vi "XW calib mesh and tree checker_PN.vi"() -> ()   [LabVIEW 2010]
uses:
  <vilib>/Utility/miscctls.llb/LVBoundsTypeDef.ctl
  Trimmed down TreeNode2D.ctl
panel:
  out "Status":string="Status report will be presented here"
  out "Null-zone check (ensure there are no gray areas within the triangle mesh)":picture
  in  "Viewport size (pix)":u32=720
  in  "Highlight mesh and tree":bool=TRUE
  out "Tri-mesh":picture
  out "Interactive mode ready":bool
  out "E2 (Volts)":dbl
  out "E1 (Volts)":dbl
  out "V (m/s)":dbl=nan
  out "U (m/s)":dbl=nan
  out "Voltages are inside calibrated region":bool
  in  "Stop interactive mode":bool
  out "Tree":picture
  out "Node stack size history":i32[](graph)
  out "All nodes processed and processed without error":bool
  in  "Sf":dbl=0.6
  in  "dq":dbl=0.3927
  in  "L0":dbl=1.0
  in  "Pad":dbl=1.01
  in  "XW_Calib_Map file path (dialog if empty)":path=path "C:/Documents and Settings/Paul Nathan/Desktop/XW Calib Map/XW Calib Map TRIMESH vi/XW_Map_Wire001OH65_080210.txt"
  # "Paul Nathan 07/03/10"
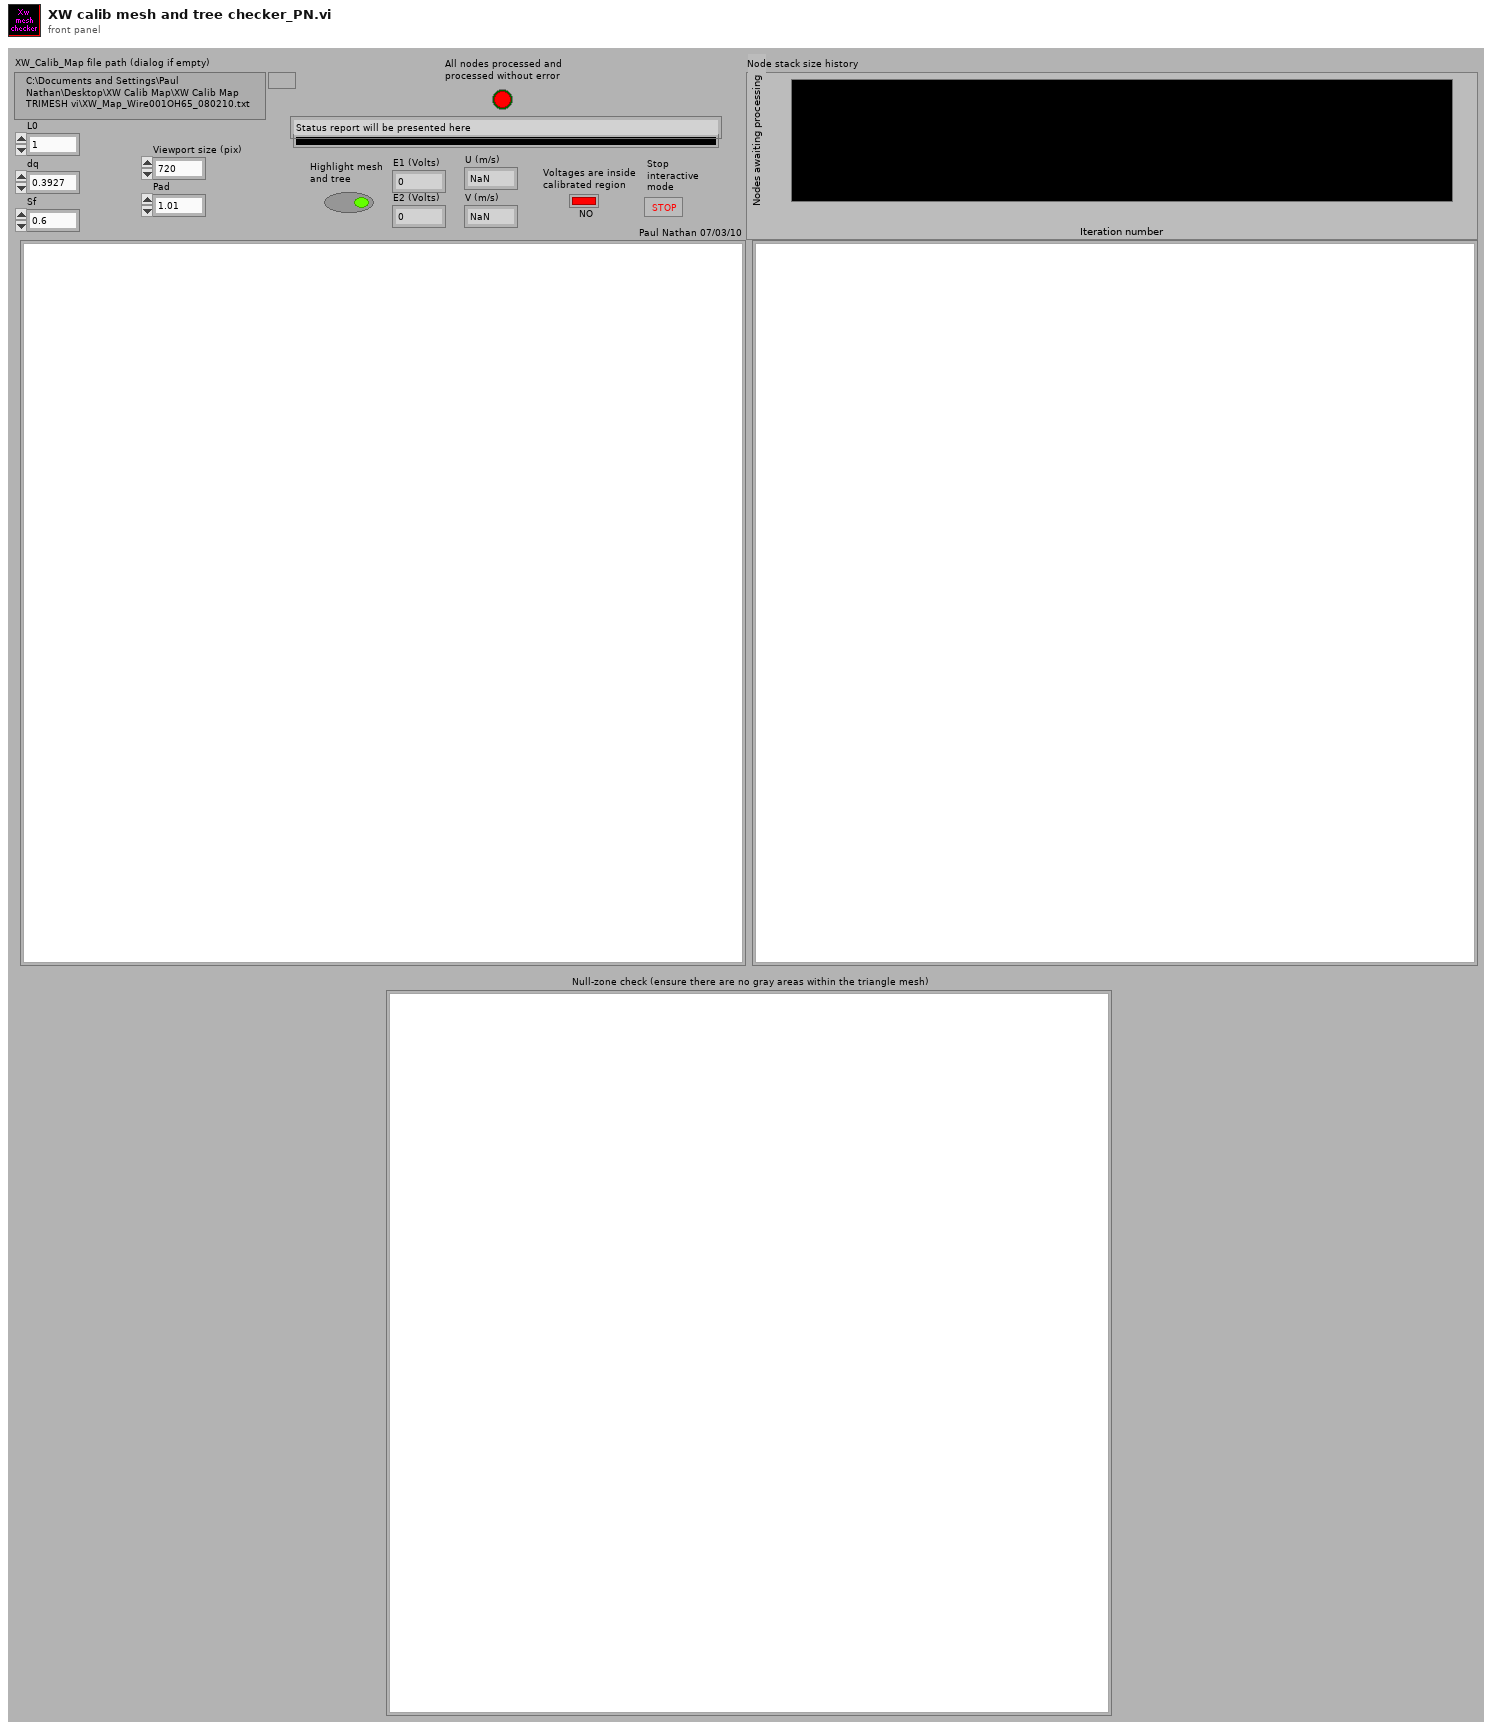
[diagram p1: front panel]
types:
  T1 = typedef "LVBoundsTypeDef.ctl" = cluster{"Width":u32, "Height":u32}
  T2 = cluster{"Width":i16, "Style":enum32{"Solid", "Dash", "Dot", "DashDot", "DashDotDot"}}
  T3 = cluster{"Width":u16, "Style":enum32{"Solid", "Dash", "Dot", "DashDot", "DashDotDot"}}
  T4 = typedef "Trimmed down TreeNode2D.ctl" = cluster{"Xmax":dbl, "Xmin":dbl, "Ymax":dbl, "Ymin":dbl, "Xc":dbl, "Yc":dbl, "ObjIndexList":i32[], "NodeQ1Index":i32, "NodeQ2Index":i32, "NodeQ3Index":i32, "NodeQ4Index":i32}
  T5 = typedef "Triangle2D.ctl" = cluster{"V10":dbl[], "V20":dbl[], "1/det":dbl, "V0":cluster{"PosVector":dbl[], "ValueVector":dbl[]}, "V1":cluster{"PosVector":dbl[], "ValueVector":dbl[]}, "V2":cluster{"PosVector":dbl[], "ValueVector":dbl[]}, "V21":dbl[]}
  T6 = cluster{"Xmax":dbl, "Xmin":dbl, "Ymax":dbl, "Ymin":dbl}
  T7 = typedef "TreeNode2D.ctl" = cluster{"Xmax":dbl, "Xmin":dbl, "Ymax":dbl, "Ymin":dbl, "Xc":dbl, "Yc":dbl, "Px":dbl, "Py":dbl, "q":dbl, "Level":i32, "ObjIndexList":i32[], "ParentIndex":i32, "NodeQ1Index":i32, "NodeQ2Index":i32, "NodeQ3Index":i32, "NodeQ4Index":i32, "EdgeVectorsQ1":dbl[][], "EdgeVectorsQ2":dbl[][], "EdgeVectorsQ3":dbl[][], "EdgeVectorsQ4":dbl[][], "PointOnEdgeVectorsQ1":dbl[][], "PointOnEdgeVectorsQ2":dbl[][], "PointOnEdgeVectorsQ3":dbl[][], "PointOnEdgeVectorsQ4":dbl[][]}
  T8 = typedef "LVMouseTypeDef.ctl" = cluster{"Mouse Position":cluster{"X":i32, "Y":i32}, "Mouse Modifiers":cluster{"Button Down":bool, "Shift Mod":bool, "Menu Mod":bool, "Option Mod":bool}}
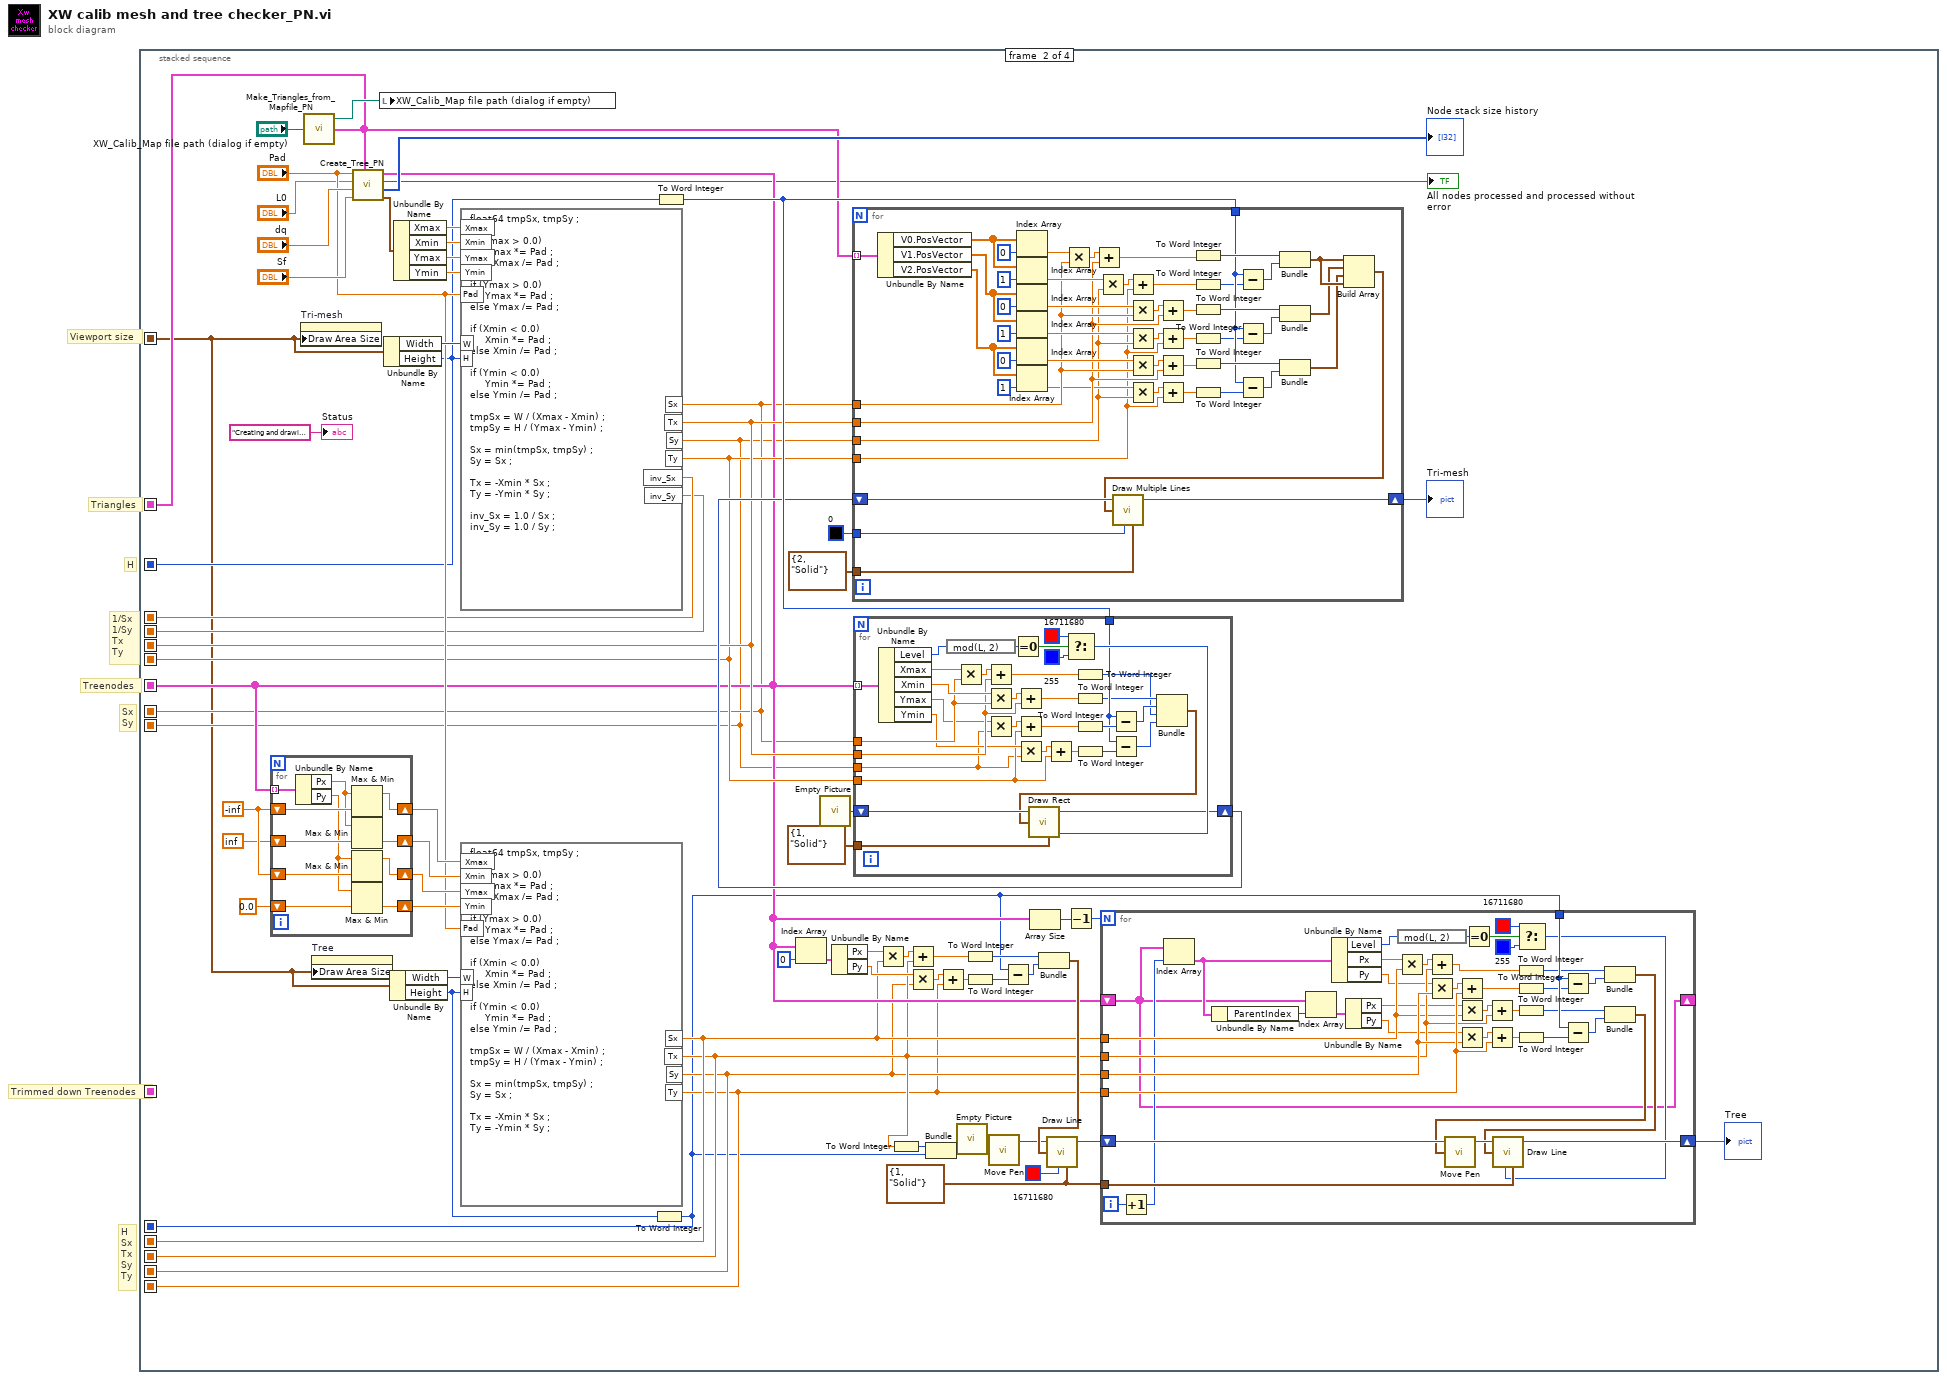
[diagram p0: block diagram]
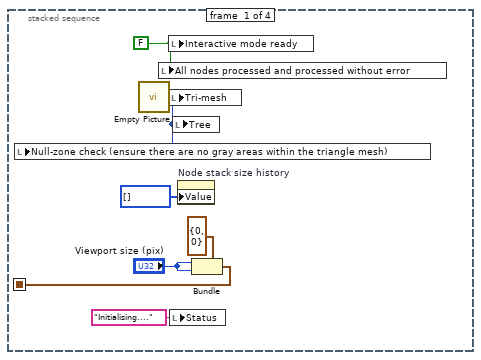
[diagram p2: hidden frame]
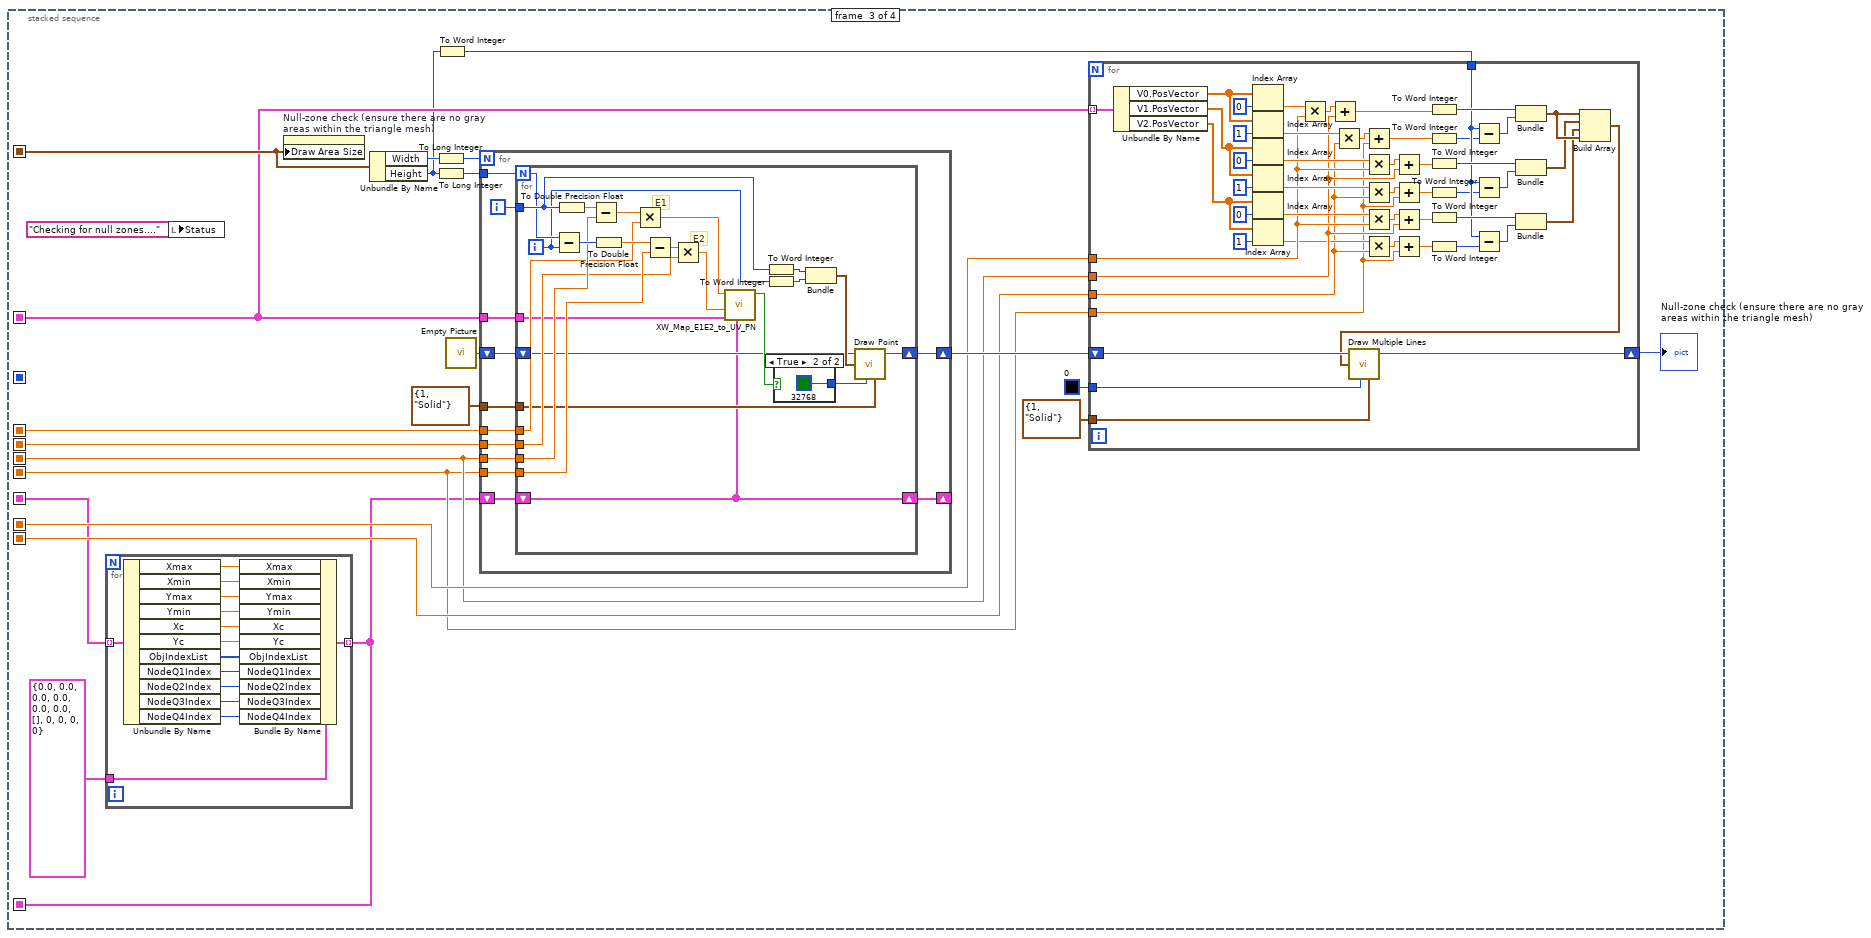
[diagram p3: hidden frame]
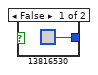
[diagram p4: hidden frame]
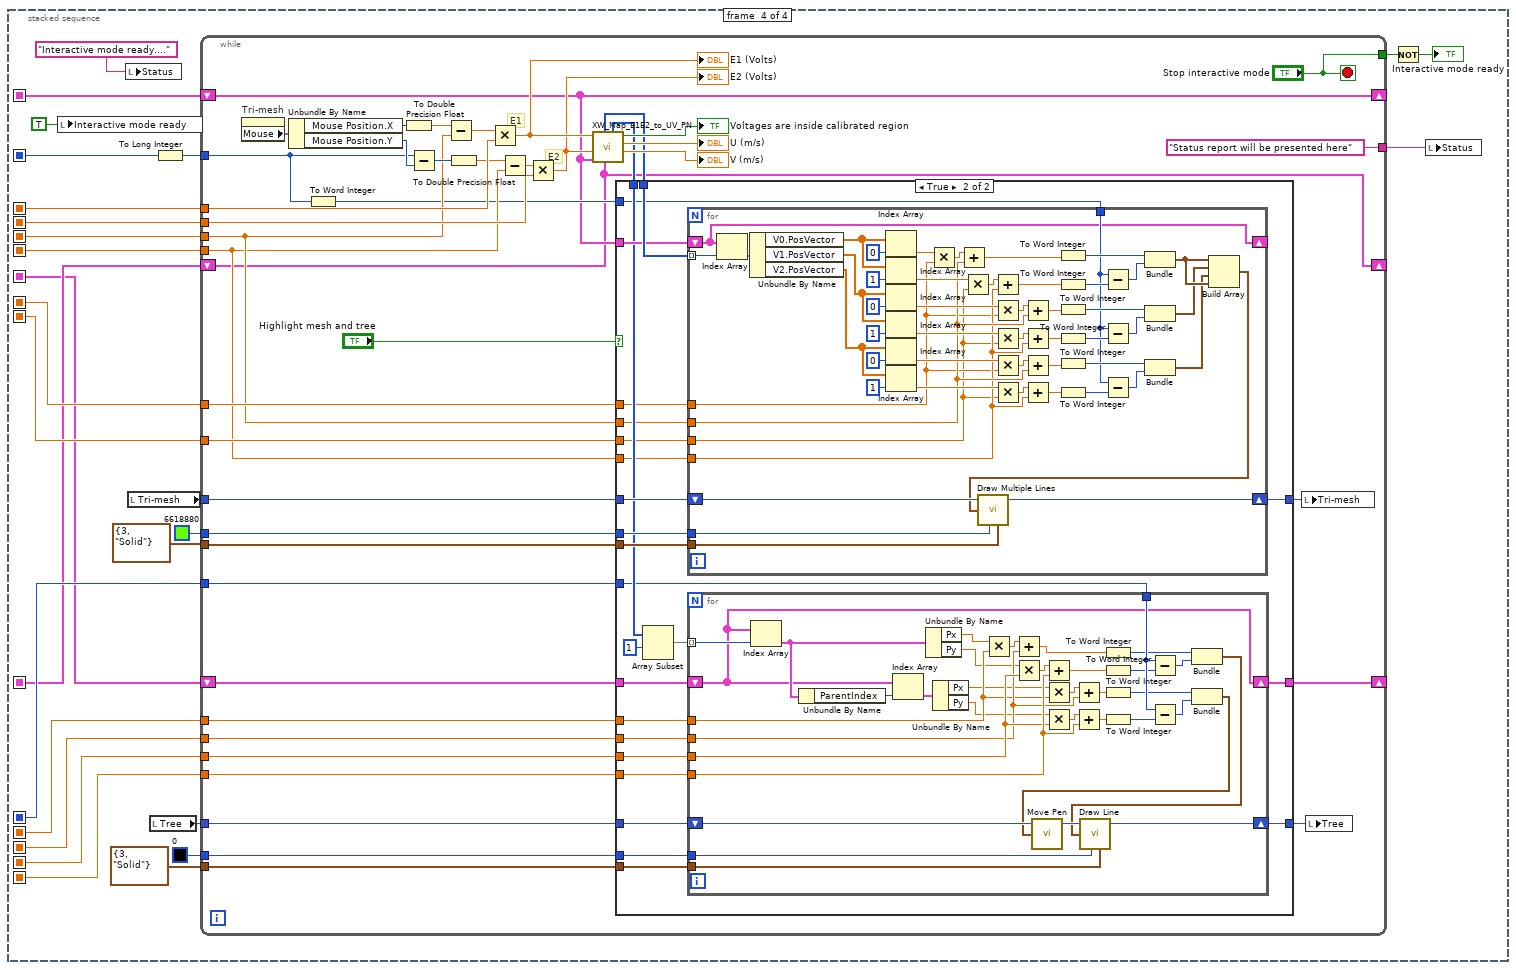
[diagram p5: hidden frame]
diagram:
  # "Trimmed down Treenodes"
  # "Viewport size"
  # "H\nSx\nTx\nSy\nTy"
  # "Sx\nSy"
  # "Treenodes"
  # "Triangles"
  # "H"
  # "1/Sx\n1/Sy\nTx\nTy"
  n1 = stacked-sequence {
    seq-local: [_ w29 _ _] -> [_ _ w230 w354]
    seq-local: [_ w28 _ _] -> [_ _ w229 w353]
    seq-local: [_ w27 _ _] -> [_ _ w219 w363]
    seq-local: [_ w26 _ _] -> [_ _ w218 w362]
    seq-local: [_ w25 _ _] -> [_ _ _ w361]
    seq-local: [_ w22 _ _] -> [_ _ w213 w337]
    seq-local: [_ w24 _ _] -> [_ _ w222 w359]
    seq-local: [_ w19 _ _] -> [_ _ w221 w348]
    seq-local: [_ w18 _ _] -> [_ _ w220 w347]
    seq-local: [_ w12 _ _] -> [_ _ _ w342]
    seq-local: [_ w16 _ _] -> [_ _ _ w346]
    seq-local: [_ w15 _ _] -> [_ _ _ w345]
    seq-local: [_ w14 _ _] -> [_ _ _ w344]
    seq-local: [_ w13 _ _] -> [_ _ _ w343]
    seq-local: [w4 _ _ _] -> [_ w11 w234 _]
    seq-local: [_ _ w212 _] -> [_ _ _ w338]
    frame #0 {
      w2 = FALSE
      n2 = call "Empty Picture"() -> ("empty picture"=w3:picture)
      n3 = local write "Null-zone check (ensure there are no gray areas within the triangle mesh)"(w3) -> ()
      n4 = local write "All nodes processed and processed without error"(w2) -> ()
      n5 = local write "Interactive mode ready"(w2) -> ()
      n6 = local write "Tri-mesh"(w3) -> ()
      n7 = local write "Status"("Initialising....") -> ()
      n8 = local write "Tree"(w3) -> ()
      n9 = property on="Node stack size history" class="WFGraph (strict)"("Value"=i32[] [] ("Node stack size history")) -> ()  [unwired: 2 in, 2 out]
      n10 = Bundle(cluster=T1 {"Width"=0, "Height"=0} ("Draw Area Size"), "Width"="Viewport size (pix)", "Height"="Viewport size (pix)") -> (w4:T1)
    }
    frame #1 {
      w32 = T3 {"Width"=1, "Style"=enum."Solid"} ("pen")
      w53 = -inf
      n11 = property on="Tri-mesh" class="Pict"("Draw Area Size"=w11) -> ()  [unwired: 2 in, 2 out]
      n12 = call "Make_Triangles_from_Mapfile_PN.vi"("XW_Calib_Map file path (dialog if empty)"="XW_Calib_Map file path (dialog if empty)") -> ("XW_Calib_Map file path"=w74:path, "Triangles"=w24:T5[])  [unwired: 1 out]
      n13 = property on="Tree" class="Pict"("Draw Area Size"=w11) -> ()  [unwired: 2 in, 2 out]
      n14 = call "Create_Tree_PN.vi"("Triangles"=w24, "Sf"="Sf", "dq"="dq", "L0"="L0", "Pad"="Pad") -> ("Mesh bounds"=w8:T6, "Node stack size history"=→"Node stack size history":i32[], "All nodes processed and processed without error"=→"All nodes processed and processed without error":bool, "TreeNodes out"=w22:T7[])
      n15 = for {
        shift-right: [w127] -> w55
        shift-left: w53 -> [w125]
        shift-right: [w126] -> w57
        shift-left: w53 -> [w124]
        shift-right: [w122] -> w56
        shift-left: inf -> [w123]
        shift-right: [w120] -> w58
        shift-left: 0.0 -> [w121]
        tunnel: w22 -> [w118] mode=indexing
        n16 = Unbundle By Name(w118) -> ("Px"=w119:dbl, "Py"=w117:dbl)
        n17 = Max & Min(x=w119, y=w125) -> (max(x,y)=w127:dbl)  [unwired: 1 out]
        n18 = Max & Min(x=w119, y=w123) -> (min(x,y)=w122:dbl)  [unwired: 1 out]
        n19 = Max & Min(x=w117, y=w124) -> (max(x,y)=w126:dbl)  [unwired: 1 out]
        n20 = Max & Min(x=w117, y=w121) -> (min(x,y)=w120:dbl)  [unwired: 1 out]
      }
      n21 = local write "XW_Calib_Map file path (dialog if empty)"(w74) -> ()
      n22 = Unbundle By Name(w11) -> ("Width"=w70:u32, "Height"=w25:u32)
      n23 = Unbundle By Name(w11) -> ("Width"=w59:u32, "Height"=w17:u32)
      n24 = Unbundle By Name(w8) -> ("Xmax"=w67:dbl, "Xmin"=w66:dbl, "Ymax"=w65:dbl, "Ymin"=w64:dbl)
      n25 = formula code="float64 tmpSx, tmpSy ;\n\nif (Xmax > 0.0)\n     Xmax *= Pad ;\nelse Xmax /= Pad ;\n\nif (Ymax > 0.0)\n     Ymax *= Pad ;\nelse Ymax /= Pad ;\n\nif (Xmin < 0.0)\n     Xmin *= Pad ;\nelse Xmin /= Pad ;\n\nif (Ymin < 0.0)\n     Ymin *= Pad ;\nelse Ymin /= Pad ;\n\ntmpSx = W / (Xmax - Xmin) ;\ntmpSy = H / (Ymax - Ymin) ;\n\nSx = min(tmpSx, tmpSy) ;\nSy = Sx ;\n\nTx = -Xmin * Sx ;\nTy = -Ymin * Sy ;\n\ninv_Sx = 1.0 / Sx ;\ninv_Sy = 1.0 / Sy ;"("Xmax"=w67, "Xmin"=w66, "Ymax"=w65, "Ymin"=w64, "W"=w70, "H"=w25, "Pad"="Pad") -> ("Sx"=w19:dbl, "Sy"=w18:dbl, "Tx"=w27:dbl, "Ty"=w26:dbl, "inv_Sx"=w29:dbl, "inv_Sy"=w28:dbl)
      n26 = formula code="float64 tmpSx, tmpSy ;\n\nif (Xmax > 0.0)\n     Xmax *= Pad ;\nelse Xmax /= Pad ;\n\nif (Ymax > 0.0)\n     Ymax *= Pad ;\nelse Ymax /= Pad ;\n\nif (Xmin < 0.0)\n     Xmin *= Pad ;\nelse Xmin /= Pad ;\n\nif (Ymin < 0.0)\n     Ymin *= Pad ;\nelse Ymin /= Pad ;\n\ntmpSx = W / (Xmax - Xmin) ;\ntmpSy = H / (Ymax - Ymin) ;\n\nSx = min(tmpSx, tmpSy) ;\nSy = Sx ;\n\nTx = -Xmin * Sx ;\nTy = -Ymin * Sy ;"("Xmax"=w55, "Xmin"=w56, "Ymax"=w57, "Ymin"=w58, "W"=w59, "H"=w17, "Pad"="Pad") -> ("Sx"=w16:dbl, "Sy"=w14:dbl, "Tx"=w15:dbl, "Ty"=w13:dbl)
      n27 = To Word Integer(number=w17) -> (16bit integer=w12:i16)
      n28 = To Word Integer(number=w25) -> (16bit integer=w61:i16)
      n29 = Index Array(array=w22, index=0) -> (element=w48:T7)
      n30 = call "Empty Picture"() -> ("empty picture"=w63:picture)
      n31 = Unbundle By Name(w48) -> ("Px"=w43:dbl, "Py"=w41:dbl)
      n32 = for {
        tunnel: w22 -> [w161] mode=indexing
        tunnel: w19 -> [w146]
        tunnel: w27 -> [w145]
        tunnel: w18 -> [w134]
        tunnel: w26 -> [w136]
        shift-right: [w152] -> w60
        shift-left: w63 -> [w155]
        tunnel: T2 {"Width"=1, "Style"=enum."Solid"} ("pen") -> [w153]
        tunnel: w61 -> [w139]
        n33 = Unbundle By Name(w161) -> ("Level"=w160:i32, "Xmax"=w150:dbl, "Xmin"=w147:dbl, "Ymax"=w142:dbl, "Ymin"=w137:dbl)
        n34 = expression code="mod(L, 2)"(w160) -> (w159:i32)
        n35 = Multiply(x=w150, y=w146) -> (x*y=w151:dbl)
        n36 = Add(x=w151, y=w145) -> (x+y=w149:dbl)
        n37 = Multiply(x=w147, y=w146) -> (x*y=w148:dbl)
        n38 = Multiply(x=w142, y=w134) -> (x*y=w143:dbl)
        n39 = Equal To 0?(x=w159) -> (x = 0?=w158:bool)
        n40 = Add(x=w148, y=w145) -> (x+y=w144:dbl)
        n41 = Add(x=w143, y=w136) -> (x+y=w141:dbl)
        n42 = Multiply(x=w137, y=w134) -> (x*y=w135:dbl)
        n43 = Add(x=w135, y=w136) -> (x+y=w133:dbl)
        n44 = Select(t=u32 16711680, s=w158, f=u32 255) -> (s? t:f=w154:u32)
        n45 = To Word Integer(number=w149) -> (16bit integer=w130:i16)
        n46 = To Word Integer(number=w144) -> (16bit integer=w132:i16)
        n47 = To Word Integer(number=w141) -> (16bit integer=w140:i16)
        n48 = To Word Integer(number=w133) -> (16bit integer=w138:i16)
        n49 = Subtract(x=w139, y=w140) -> (x-y=w131:i16)
        n50 = Subtract(x=w139, y=w138) -> (x-y=w129:i16)
        n51 = Bundle(w132, w131, w130, w129) -> (w128:cluster{i16, i16, i16, i16})  [unwired: 1 out]
        n52 = call <vilib>:"Draw Rect.vi"("picture"=w155, "rect"=w128, "color(black)"=w154, "pen"=w153) -> ("new picture"=w152:picture)  [unwired: 1 in, 4 out]
      }
      n53 = for {
        tunnel: w24 -> [w211] mode=indexing
        shift-right: [w207] -> w23
        shift-left: w60 -> [w208]
        tunnel: u32 0 -> [w210]
        tunnel: T3 {"Width"=2, "Style"=enum."Solid"} ("pen") -> [w209]
        tunnel: w19 -> [w184]
        tunnel: w27 -> [w183]
        tunnel: w18 -> [w180]
        tunnel: w26 -> [w179]
        tunnel: w61 -> [w168]
        n54 = Unbundle By Name(w211) -> ("V0.PosVector"=w197:dbl[], "V1.PosVector"=w196:dbl[], "V2.PosVector"=w195:dbl[])
        n55 = Index Array(array=w197, index=0) -> (element=w194:dbl)
        n56 = Index Array(array=w197, index=1) -> (element=w191:dbl)
        n57 = Index Array(array=w196, index=0) -> (element=w189:dbl)
        n58 = Index Array(array=w196, index=1) -> (element=w187:dbl)
        n59 = Index Array(array=w195, index=0) -> (element=w185:dbl)
        n60 = Index Array(array=w195, index=1) -> (element=w181:dbl)
        n61 = Multiply(x=w194, y=w184) -> (x*y=w193:dbl)
        n62 = Add(x=w193, y=w183) -> (x+y=w175:dbl)
        n63 = Multiply(x=w191, y=w180) -> (x*y=w192:dbl)
        n64 = Add(x=w192, y=w179) -> (x+y=w174:dbl)
        n65 = Multiply(x=w189, y=w184) -> (x*y=w190:dbl)
        n66 = Multiply(x=w187, y=w180) -> (x*y=w188:dbl)
        n67 = Multiply(x=w185, y=w184) -> (x*y=w186:dbl)
        n68 = Multiply(x=w181, y=w180) -> (x*y=w182:dbl)
        n69 = Add(x=w190, y=w183) -> (x+y=w173:dbl)
        n70 = Add(x=w188, y=w179) -> (x+y=w172:dbl)
        n71 = Add(x=w186, y=w183) -> (x+y=w171:dbl)
        n72 = Add(x=w182, y=w179) -> (x+y=w170:dbl)
        n73 = To Word Integer(number=w175) -> (16bit integer=w178:i16)
        n74 = To Word Integer(number=w174) -> (16bit integer=w167:i16)
        n75 = To Word Integer(number=w173) -> (16bit integer=w177:i16)
        n76 = To Word Integer(number=w172) -> (16bit integer=w166:i16)
        n77 = To Word Integer(number=w171) -> (16bit integer=w176:i16)
        n78 = To Word Integer(number=w170) -> (16bit integer=w165:i16)
        n79 = Subtract(x=w168, y=w167) -> (x-y=w164:i16)
        n80 = Subtract(x=w168, y=w166) -> (x-y=w163:i16)
        n81 = Subtract(x=w168, y=w165) -> (x-y=w162:i16)
        n82 = Bundle(w178, w164) -> (w204:cluster{i16, i16})  [unwired: 1 out]
        n83 = Bundle(w177, w163) -> (w201:cluster{i16, i16})  [unwired: 1 out]
        n84 = Bundle(w176, w162) -> (w198:cluster{i16, i16})  [unwired: 1 out]
        n85 = Build Array(w204, w201, w198, w204) -> (w169:cluster{i16, i16}[])
        n86 = call <vilib>:"Draw Multiple Lines.vi"("picture"=w208, "line endpoints"=w169, "color(black)"=w210, "pen"=w209) -> ("new picture"=w207:picture)  [unwired: 1 in, 4 out]
      }
      "Tri-mesh" <- w23
      n87 = Multiply(x=w43, y=w16) -> (x*y=w44:dbl)
      n88 = To Word Integer(number=w15) -> (16bit integer=w47:i16)
      n89 = Add(x=w44, y=w15) -> (x+y=w40:dbl)
      n90 = Multiply(x=w41, y=w14) -> (x*y=w42:dbl)
      n91 = Bundle(w47, w12) -> (w46:cluster{i16, i16})  [unwired: 1 out]
      n92 = Add(x=w42, y=w13) -> (x+y=w39:dbl)
      n93 = call "Empty Picture"() -> ("empty picture"=w45:picture)
      n94 = To Word Integer(number=w40) -> (16bit integer=w37:i16)
      n95 = To Word Integer(number=w39) -> (16bit integer=w38:i16)
      n96 = call <vilib>:"Move Pen.vi"("new position"=w46, "picture"=w45) -> ("new picture"=w34:picture)  [unwired: 1 in, 2 out]
      n97 = Subtract(x=w12, y=w38) -> (x-y=w36:i16)
      n98 = Array Size(array=w22) -> (size(s)=w21:i32)
      n99 = Bundle(w37, w36) -> (w35:cluster{i16, i16})  [unwired: 1 out]
      n100 = call <vilib>:"Draw Line.vi"("picture"=w34, "end point"=w35, "color(black)"=u32 16711680, "pen"=w32) -> ("new picture"=w31:picture)  [unwired: 1 in, 4 out]
      n101 = Decrement(x=w21) -> (x-1=w20:i32)
      n102 = for {
        N: w20 -> [_]
        shift-right: [w115] -> w30
        shift-left: w31 -> [w116]
        tunnel: w32 -> [w113]
        tunnel: w12 -> [w108]
        tunnel: w16 -> [w109]
        tunnel: w15 -> [w110]
        tunnel: w14 -> [w111]
        tunnel: w13 -> [w112]
        shift-right: [w76] -> _
        shift-left: w22 -> [w76]
        i -> [w79]
        n103 = Increment(x=w79) -> (x+1=w78:i32)
        n104 = Index Array(array=w76, index=w78) -> (element=w77:T7)
        n105 = Unbundle By Name(w77) -> ("ParentIndex"=w114:i32)
        n106 = Index Array(array=w76, index=w114) -> (element=w107:T7)
        n107 = Unbundle By Name(w77) -> ("Level"=w102:i32, "Px"=w98:dbl, "Py"=w94:dbl)
        n108 = Unbundle By Name(w107) -> ("Px"=w92:dbl, "Py"=w89:dbl)
        n109 = Multiply(x=w98, y=w109) -> (x*y=w99:dbl)
        n110 = expression code="mod(L, 2)"(w102) -> (w103:i32)
        n111 = Add(x=w99, y=w110) -> (x+y=w97:dbl)
        n112 = Multiply(x=w94, y=w111) -> (x*y=w95:dbl)
        n113 = Add(x=w95, y=w112) -> (x+y=w91:dbl)
        n114 = Multiply(x=w92, y=w109) -> (x*y=w93:dbl)
        n115 = Multiply(x=w89, y=w111) -> (x*y=w90:dbl)
        n116 = Equal To 0?(x=w103) -> (x = 0?=w104:bool)
        n117 = Add(x=w93, y=w110) -> (x+y=w88:dbl)
        n118 = Add(x=w90, y=w112) -> (x+y=w87:dbl)
        n119 = To Word Integer(number=w97) -> (16bit integer=w96:i16)
        n120 = To Word Integer(number=w91) -> (16bit integer=w83:i16)
        n121 = To Word Integer(number=w88) -> (16bit integer=w86:i16)
        n122 = To Word Integer(number=w87) -> (16bit integer=w82:i16)
        n123 = Select(t=u32 16711680, s=w104, f=u32 255) -> (s? t:f=w101:u32)
        n124 = Subtract(x=w108, y=w83) -> (x-y=w85:i16)
        n125 = Subtract(x=w108, y=w82) -> (x-y=w84:i16)
        n126 = Bundle(w96, w85) -> (w80:cluster{i16, i16})  [unwired: 1 out]
        n127 = Bundle(w86, w84) -> (w81:cluster{i16, i16})  [unwired: 1 out]
        n128 = call <vilib>:"Move Pen.vi"("new position"=w81, "picture"=w116) -> ("new picture"=w100:picture)  [unwired: 1 in, 2 out]
        n129 = call <vilib>:"Draw Line.vi"("picture"=w100, "end point"=w80, "color(black)"=w101, "pen"=w113) -> ("new picture"=w115:picture)  [unwired: 1 in, 4 out]
      }
      "Tree" <- w30
      "Status" <- "Creating and drawing mesh, spatial hierarchy and address tree...."
    }
    frame #2 {
      n130 = for {
        tunnel: w213 -> [w248] mode=indexing
        tunnel: [w246] -> w212 mode=indexing
        tunnel: T4 {"Xmax"=0.0, "Xmin"=0.0, "Ymax"=0.0, "Ymin"=0.0, "Xc"=0.0, "Yc"=0.0, "ObjIndexList"=[], "NodeQ1Index"=0, "NodeQ2Index"=0, "NodeQ3Index"=0, "NodeQ4Index"=0} ("Trimmed down TreeNode") -> [w247]
        n131 = Unbundle By Name(w248) -> ("Xmax"=w245:dbl, "Xmin"=w244:dbl, "Ymax"=w243:dbl, "Ymin"=w242:dbl, "Xc"=w241:dbl, "Yc"=w240:dbl, "ObjIndexList"=w239:i32[], "NodeQ1Index"=w238:i32, "NodeQ2Index"=w237:i32, "NodeQ3Index"=w236:i32, "NodeQ4Index"=w235:i32)
        n132 = Bundle By Name(cluster=w247, "Xmax"=w245, "Xmin"=w244, "Ymax"=w243, "Ymin"=w242, "Xc"=w241, "Yc"=w240, "ObjIndexList"=w239, "NodeQ1Index"=w238, "NodeQ2Index"=w237, "NodeQ3Index"=w236, "NodeQ4Index"=w235) -> (w246:T4)
      }
      n133 = local write "Status"("Checking for null zones....") -> ()
      n134 = property on="Null-zone check (ensure there are no gray areas within the triangle mesh)" class="Pict"("Draw Area Size"=w234) -> ()  [unwired: 2 in, 2 out]
      n135 = Unbundle By Name(w234) -> ("Width"=w232:u32, "Height"=w217:u32)
      n136 = To Long Integer(number=w232) -> (32bit integer=w231:i32)
      n137 = To Long Integer(number=w217) -> (32bit integer=w233:i32)
      n138 = To Word Integer(number=w217) -> (16bit integer=w216:i16)
      n139 = call "Empty Picture"() -> ("empty picture"=w227:picture)
      n140 = for {
        N: w231 -> [_]
        tunnel: w233 -> [w305]
        tunnel: w230 -> [w310]
        tunnel: w229 -> [w309]
        tunnel: w219 -> [w308]
        tunnel: w218 -> [w307]
        tunnel: w222 -> [w303]
        tunnel: T3 {"Width"=1, "Style"=enum."Solid"} ("pen") -> [w302]
        shift-right: [w300] -> w223
        shift-left: w227 -> [w301]
        shift-right: [w299] -> _
        shift-left: w212 -> [w304]
        i -> [w306]
        n141 = for {
          N: w305 -> [w321]
          tunnel: w310 -> [w327]
          tunnel: w309 -> [w326]
          tunnel: w308 -> [w329]
          tunnel: w307 -> [w328]
          tunnel: w306 -> [w322]
          tunnel: w303 -> [w323]
          tunnel: w302 -> [w320]
          shift-right: [w319] -> w300
          shift-left: w301 -> [w313]
          shift-right: [w311] -> w299
          shift-left: w304 -> [w311]
          i -> [w312]
          # "E2"
          # "E1"
          n142 = Subtract(x=w321, y=w312) -> (x-y=w332:i32)
          n143 = To Double Precision Float(number=w322) -> (double precision float=w334:dbl)
          n144 = Subtract(x=w334, y=w329) -> (x-y=w333:dbl)
          n145 = To Double Precision Float(number=w332) -> (double precision float=w331:dbl)
          n146 = Multiply(x=w333, y=w327) -> (x*y=w325:dbl)
          n147 = Subtract(x=w331, y=w328) -> (x-y=w330:dbl)
          n148 = Multiply(x=w330, y=w326) -> (x*y=w324:dbl)
          n149 = call "XW_Map_E1E2_to_UV_PN.vi"("Trimmed down TreeNode array"=w311, "Triangulated XW Calib Map Mesh"=w323, "(E2 / G2) + O2 (Volts)"=w324, "(E1 / G1) + O1 (Volts)"=w325) -> ("Voltages are inside calibrated region"=w315:bool)  [unwired: 7 out]
          n150 = To Word Integer(number=w322) -> (16bit integer=w318:i16)
          n151 = To Word Integer(number=w312) -> (16bit integer=w317:i16)
          n152 = case shown="True" w315 {
            tunnel: [u32 13816530 u32 32768] -> w314
            frame False {
            }
            frame True {
            }
          }
          n153 = Bundle(w318, w317) -> (w316:cluster{i16, i16})  [unwired: 1 out]
          n154 = call <vilib>:"Draw Point.vi"("picture"=w313, "point(x,y)"=w316, "color(black)"=w314, "pen"=w320) -> ("new picture"=w319:picture)  [unwired: 5 out]
        }
      }
      n155 = for {
        tunnel: w222 -> [w298] mode=indexing
        shift-right: [w294] -> w224
        shift-left: w223 -> [w295]
        tunnel: u32 0 -> [w297]
        tunnel: T3 {"Width"=1, "Style"=enum."Solid"} ("pen") -> [w296]
        tunnel: w221 -> [w271]
        tunnel: w219 -> [w270]
        tunnel: w220 -> [w267]
        tunnel: w218 -> [w266]
        tunnel: w216 -> [w255]
        n156 = Unbundle By Name(w298) -> ("V0.PosVector"=w284:dbl[], "V1.PosVector"=w283:dbl[], "V2.PosVector"=w282:dbl[])
        n157 = Index Array(array=w284, index=0) -> (element=w281:dbl)
        n158 = Index Array(array=w284, index=1) -> (element=w278:dbl)
        n159 = Index Array(array=w283, index=0) -> (element=w276:dbl)
        n160 = Index Array(array=w283, index=1) -> (element=w274:dbl)
        n161 = Index Array(array=w282, index=0) -> (element=w272:dbl)
        n162 = Index Array(array=w282, index=1) -> (element=w268:dbl)
        n163 = Multiply(x=w281, y=w271) -> (x*y=w280:dbl)
        n164 = Add(x=w280, y=w270) -> (x+y=w262:dbl)
        n165 = Multiply(x=w278, y=w267) -> (x*y=w279:dbl)
        n166 = Add(x=w279, y=w266) -> (x+y=w261:dbl)
        n167 = Multiply(x=w276, y=w271) -> (x*y=w277:dbl)
        n168 = Multiply(x=w274, y=w267) -> (x*y=w275:dbl)
        n169 = Multiply(x=w272, y=w271) -> (x*y=w273:dbl)
        n170 = Multiply(x=w268, y=w267) -> (x*y=w269:dbl)
        n171 = Add(x=w277, y=w270) -> (x+y=w260:dbl)
        n172 = Add(x=w275, y=w266) -> (x+y=w259:dbl)
        n173 = Add(x=w273, y=w270) -> (x+y=w258:dbl)
        n174 = Add(x=w269, y=w266) -> (x+y=w257:dbl)
        n175 = To Word Integer(number=w262) -> (16bit integer=w265:i16)
        n176 = To Word Integer(number=w261) -> (16bit integer=w254:i16)
        n177 = To Word Integer(number=w260) -> (16bit integer=w264:i16)
        n178 = To Word Integer(number=w259) -> (16bit integer=w253:i16)
        n179 = To Word Integer(number=w258) -> (16bit integer=w263:i16)
        n180 = To Word Integer(number=w257) -> (16bit integer=w252:i16)
        n181 = Subtract(x=w255, y=w254) -> (x-y=w251:i16)
        n182 = Subtract(x=w255, y=w253) -> (x-y=w250:i16)
        n183 = Subtract(x=w255, y=w252) -> (x-y=w249:i16)
        n184 = Bundle(w265, w251) -> (w291:cluster{i16, i16})  [unwired: 1 out]
        n185 = Bundle(w264, w250) -> (w288:cluster{i16, i16})  [unwired: 1 out]
        n186 = Bundle(w263, w249) -> (w285:cluster{i16, i16})  [unwired: 1 out]
        n187 = Build Array(w291, w288, w285, w291) -> (w256:cluster{i16, i16}[])
        n188 = call <vilib>:"Draw Multiple Lines.vi"("picture"=w295, "line endpoints"=w256, "color(black)"=w297, "pen"=w296) -> ("new picture"=w294:picture)  [unwired: 1 in, 4 out]
      }
      "Null-zone check (ensure there are no gray areas within the triangle mesh)" <- w224
    }
    frame #3 {
      n189 = local write "Interactive mode ready"(TRUE ("Interactive mode ready")) -> ()
      n190 = local write "Status"("Interactive mode ready....") -> ()
      n191 = local read "Tri-mesh"() -> (w352:picture)
      n192 = local read "Tree"() -> (w351:picture)
      n193 = To Long Integer(number=w361) -> (32bit integer=w360:i32)
      n194 = while {
        tunnel: w354 -> [w403]
        tunnel: w353 -> [w400]
        tunnel: w363 -> [w381]
        tunnel: w362 -> [w379]
        tunnel: w360 -> [w378]
        tunnel: ["Stop interactive mode"] -> w357
        tunnel: u32 6618880 -> [w392]
        tunnel: T3 {"Width"=3, "Style"=enum."Solid"} ("pen") -> [w391]
        tunnel: w348 -> [w382]
        tunnel: w347 -> [w380]
        tunnel: w352 -> [w388]
        tunnel: w351 -> [w386]
        tunnel: u32 0 -> [w385]
        tunnel: T3 {"Width"=3, "Style"=enum."Solid"} ("pen") -> [w384]
        tunnel: w346 -> [w376]
        tunnel: w345 -> [w375]
        tunnel: w344 -> [w374]
        tunnel: w343 -> [w373]
        tunnel: w342 -> [w372]
        tunnel: ["Status report will be presented here"] -> w339
        shift-right: [w367] -> _
        shift-left: w359 -> [w367]
        shift-right: [w365] -> _
        shift-left: w337 -> [w366]
        shift-right: [w364] -> _
        shift-left: w338 -> [w364]
        stop <- "Stop interactive mode" stop-if-true
        # "E2"
        # "E1"
        n195 = property on="Tri-mesh" class="Pict"() -> ("Mouse"=w393:T8)  [unwired: 2 in, 2 out]
        n196 = Unbundle By Name(w393) -> ("Mouse Position.X"=w406:i32, "Mouse Position.Y"=w402:i32)
        n197 = To Word Integer(number=w378) -> (16bit integer=w377:i16)
        n198 = To Double Precision Float(number=w406) -> (double precision float=w405:dbl)
        n199 = Subtract(x=w378, y=w402) -> (x-y=w401:i32)
        n200 = Subtract(x=w405, y=w381) -> (x-y=w404:dbl)
        n201 = To Double Precision Float(number=w401) -> (double precision float=w399:dbl)
        n202 = Multiply(x=w404, y=w403) -> (x*y=w390:dbl)
        "E1 (Volts)" <- w390
        n203 = Subtract(x=w399, y=w379) -> (x-y=w398:dbl)
        n204 = Multiply(x=w398, y=w400) -> (x*y=w389:dbl)
        "E2 (Volts)" <- w389
        n205 = call "XW_Map_E1E2_to_UV_PN.vi"("Trimmed down TreeNode array"=w364, "Triangulated XW Calib Map Mesh"=w367, "(E2 / G2) + O2 (Volts)"=w389, "(E1 / G1) + O1 (Volts)"=w390) -> ("V (m/s)"=→"V (m/s)":dbl, "U (m/s)"=→"U (m/s)":dbl, "Voltages are inside calibrated region"=→"Voltages are inside calibrated region":bool, "Indices of traversed treenodes"=w383:i32[], "Indices of triangle array to test fully"=w387:i32[])  [unwired: 3 out]
        n206 = case shown="True" "Highlight mesh and tree" {
          tunnel: w392 -> [_ w434]
          tunnel: w391 -> [_ w433]
          tunnel: w388 -> [w409 w432]
          tunnel: w387 -> [_ w431]
          tunnel: w367 -> [_ w430]
          tunnel: w386 -> [w408 w429]
          tunnel: w385 -> [_ w428]
          tunnel: w384 -> [_ w427]
          tunnel: w383 -> [_ w426]
          tunnel: w366 -> [w407 w425]
          tunnel: w382 -> [_ w424]
          tunnel: w381 -> [_ w423]
          tunnel: w380 -> [_ w422]
          tunnel: w379 -> [_ w421]
          tunnel: w377 -> [_ w418]
          tunnel: w376 -> [_ w417]
          tunnel: w375 -> [_ w416]
          tunnel: w374 -> [_ w415]
          tunnel: w373 -> [_ w414]
          tunnel: w372 -> [_ w413]
          tunnel: [w408 w412] -> w370
          tunnel: [w409 w411] -> w369
          tunnel: [w407 w410] -> w365
          frame False {
          }
          frame True {
            n207 = Array Subset(array=w426, index=1) -> (w420:i32[])  [unwired: 1 in]
            n208 = for {
              tunnel: w434 -> [w480]
              tunnel: w433 -> [w479]
              tunnel: w423 -> [w478]
              tunnel: w421 -> [w477]
              tunnel: w418 -> [w476]
              tunnel: w424 -> [w475]
              tunnel: w422 -> [w474]
              tunnel: w431 -> [w473] mode=indexing
              shift-right: [w471] -> w411
              shift-left: w432 -> [w521]
              shift-right: [w470] -> _
              shift-left: w430 -> [w470]
              n209 = Index Array(array=w470, index=w473) -> (element=w472:T5)
              n210 = Unbundle By Name(w472) -> ("V0.PosVector"=w511:dbl[], "V1.PosVector"=w510:dbl[], "V2.PosVector"=w509:dbl[])
              n211 = Index Array(array=w511, index=0) -> (element=w508:dbl)
              n212 = Index Array(array=w511, index=1) -> (element=w505:dbl)
              n213 = Index Array(array=w510, index=0) -> (element=w503:dbl)
              n214 = Index Array(array=w510, index=1) -> (element=w501:dbl)
              n215 = Index Array(array=w509, index=0) -> (element=w499:dbl)
              n216 = Index Array(array=w509, index=1) -> (element=w497:dbl)
              n217 = Multiply(x=w508, y=w475) -> (x*y=w507:dbl)
              n218 = Add(x=w507, y=w478) -> (x+y=w493:dbl)
              n219 = Multiply(x=w505, y=w474) -> (x*y=w506:dbl)
              n220 = Add(x=w506, y=w477) -> (x+y=w492:dbl)
              n221 = Multiply(x=w503, y=w475) -> (x*y=w504:dbl)
              n222 = Multiply(x=w501, y=w474) -> (x*y=w502:dbl)
              n223 = Multiply(x=w499, y=w475) -> (x*y=w500:dbl)
              n224 = Multiply(x=w497, y=w474) -> (x*y=w498:dbl)
              n225 = Add(x=w504, y=w478) -> (x+y=w491:dbl)
              n226 = Add(x=w502, y=w477) -> (x+y=w490:dbl)
              n227 = Add(x=w500, y=w478) -> (x+y=w489:dbl)
              n228 = Add(x=w498, y=w477) -> (x+y=w488:dbl)
              n229 = To Word Integer(number=w493) -> (16bit integer=w496:i16)
              n230 = To Word Integer(number=w492) -> (16bit integer=w486:i16)
              n231 = To Word Integer(number=w491) -> (16bit integer=w495:i16)
              n232 = To Word Integer(number=w490) -> (16bit integer=w485:i16)
              n233 = To Word Integer(number=w489) -> (16bit integer=w494:i16)
              n234 = To Word Integer(number=w488) -> (16bit integer=w484:i16)
              n235 = Subtract(x=w476, y=w486) -> (x-y=w483:i16)
              n236 = Subtract(x=w476, y=w485) -> (x-y=w482:i16)
              n237 = Subtract(x=w476, y=w484) -> (x-y=w481:i16)
              n238 = Bundle(w496, w483) -> (w518:cluster{i16, i16})  [unwired: 1 out]
              n239 = Bundle(w495, w482) -> (w515:cluster{i16, i16})  [unwired: 1 out]
              n240 = Bundle(w494, w481) -> (w512:cluster{i16, i16})  [unwired: 1 out]
              n241 = Build Array(w518, w515, w512, w518) -> (w487:cluster{i16, i16}[])
              n242 = call <vilib>:"Draw Multiple Lines.vi"("picture"=w521, "line endpoints"=w487, "color(black)"=w480, "pen"=w479) -> ("new picture"=w471:picture)  [unwired: 1 in, 4 out]
            }
            n243 = for {
              shift-right: [w468] -> w412
              shift-left: w429 -> [w469]
              tunnel: w427 -> [w466]
              tunnel: w413 -> [w461]
              tunnel: w417 -> [w462]
              tunnel: w416 -> [w463]
              tunnel: w415 -> [w464]
              tunnel: w414 -> [w465]
              tunnel: w428 -> [w437]
              tunnel: w420 -> [w436] mode=indexing
              shift-right: [w435] -> w410
              shift-left: w425 -> [w435]
              n244 = Index Array(array=w435, index=w436) -> (element=w438:T7)
              n245 = Unbundle By Name(w438) -> ("ParentIndex"=w467:i32)
              n246 = Index Array(array=w435, index=w467) -> (element=w460:T7)
              n247 = Unbundle By Name(w438) -> ("Px"=w457:dbl, "Py"=w453:dbl)
              n248 = Unbundle By Name(w460) -> ("Px"=w451:dbl, "Py"=w448:dbl)
              n249 = Multiply(x=w457, y=w462) -> (x*y=w458:dbl)
              n250 = Add(x=w458, y=w463) -> (x+y=w456:dbl)
              n251 = Multiply(x=w453, y=w464) -> (x*y=w454:dbl)
              n252 = Add(x=w454, y=w465) -> (x+y=w450:dbl)
              n253 = Multiply(x=w451, y=w462) -> (x*y=w452:dbl)
              n254 = Multiply(x=w448, y=w464) -> (x*y=w449:dbl)
              n255 = Add(x=w452, y=w463) -> (x+y=w447:dbl)
              n256 = Add(x=w449, y=w465) -> (x+y=w446:dbl)
              n257 = To Word Integer(number=w456) -> (16bit integer=w455:i16)
              n258 = To Word Integer(number=w450) -> (16bit integer=w442:i16)
              n259 = To Word Integer(number=w447) -> (16bit integer=w445:i16)
              n260 = To Word Integer(number=w446) -> (16bit integer=w441:i16)
              n261 = Subtract(x=w461, y=w442) -> (x-y=w444:i16)
              n262 = Subtract(x=w461, y=w441) -> (x-y=w443:i16)
              n263 = Bundle(w455, w444) -> (w439:cluster{i16, i16})  [unwired: 1 out]
              n264 = Bundle(w445, w443) -> (w440:cluster{i16, i16})  [unwired: 1 out]
              n265 = call <vilib>:"Move Pen.vi"("new position"=w440, "picture"=w469) -> ("new picture"=w459:picture)  [unwired: 1 in, 2 out]
              n266 = call <vilib>:"Draw Line.vi"("picture"=w459, "end point"=w439, "color(black)"=w437, "pen"=w466) -> ("new picture"=w468:picture)  [unwired: 1 in, 4 out]
            }
          }
        }
        n267 = local write "Tri-mesh"(w369) -> ()
        n268 = local write "Tree"(w370) -> ()
      }
      n269 = Not(x=w357) -> (.not. x?=→"Interactive mode ready":bool)
      n270 = local write "Status"(w339) -> ()
    }
  }
